vi "GFITS_SetHdrTemplate.vi"(9 "ref path":path, 10 "path":path, 11 "Database RefNum":T1) -> ()   [LabVIEW 2016]
uses:
  DBSHAND/private/vis/DatabaseHand_RefNum.ctl
  DBSHAND/private/vis/DatabaseHand_Element_Set(path).vi
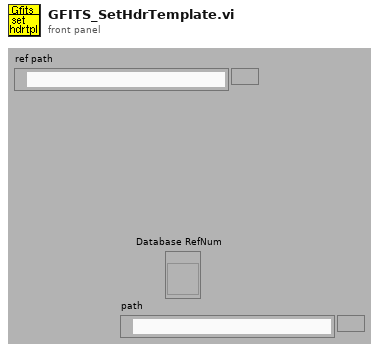
[diagram p1: front panel]
types:
  T1 = typedef "DatabaseHand_RefNum.ctl" = refnum<vi>
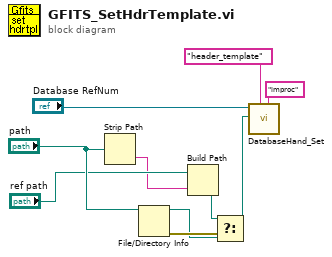
[diagram p0: block diagram]
diagram:
  n1 = Strip Path(path="path") -> (name=w2:string)  [unwired: 1 out]
  n2 = File/Directory Info(path="path") -> (path out=w6:path, error out=w7:errorcluster)  [unwired: 1 in, 5 out]
  n3 = Build Path(base path="ref path", name or relative path=w2) -> (appended path=w1:path)
  n4 = Select(t=w1, s=w7, f=w6) -> (s? t:f=w5:path)
  n5 = call-poly "DatabaseHand_Set.vi"("group"="improc", "name"="header_template", "value"=w5, "Database RefNum in"="Database RefNum") -> ()  [unwired: 4 in, 4 out]
